vi "client.vi"() -> ()   [LabVIEW 2020]
uses:
  <vilib>/httpClient/LabVIEWHTTPClient.lvlib
panel:
  out "Output":picture
  out "Selected Image":picture
  in  "Path":path
  out "body":string
  in  "Server Address":string
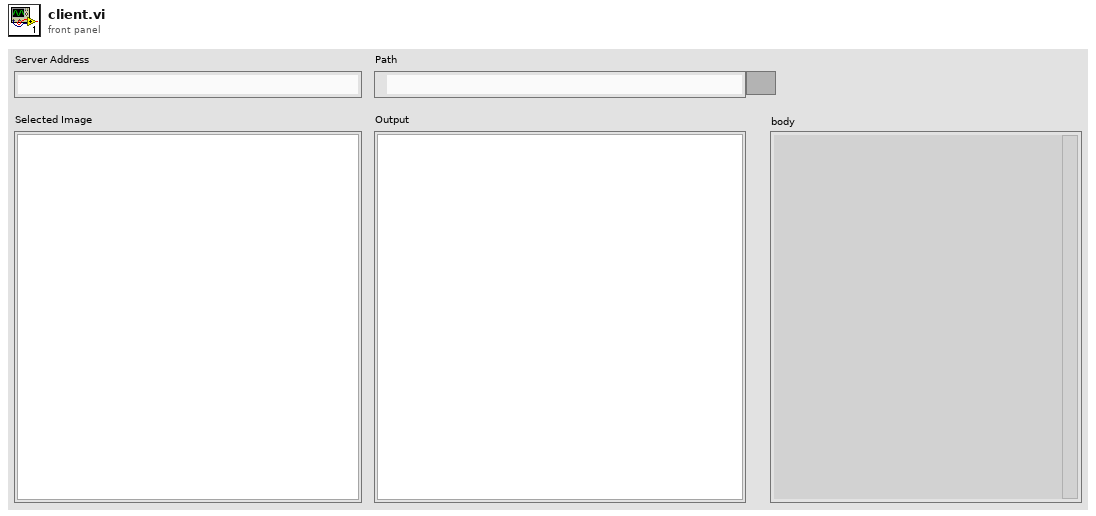
[diagram p1: front panel]
types:
  T1 = typedef "imagedata.ctl" = cluster{"image type":i32, "image depth":i32, "image":u8[], "mask":u8[], "colors":u32[], "Rectangle":cluster{"left":i16, "top":i16, "right":i16, "bottom":i16}}
  T2 = cluster{"Name":string, string, "Path":path, "name":string, string}
  T3 = cluster{"Name":string, string, "Path":path, "name":string, string}[]
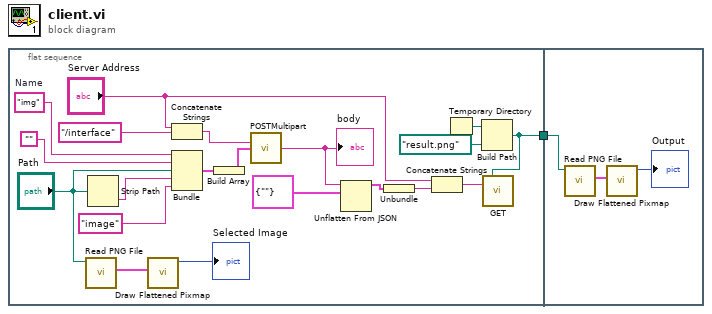
[diagram p0: block diagram]
diagram:
  n1 = flat-sequence {
    tunnel: [w3] -> w1
    tunnel: w1 -> [w22]
    frame #0 {
      w6 = "img"  # Name
      n2 = call <vilib>:"Read PNG File.vi"("path to PNG file"="Path") -> ("image data"=w14:T1)  [unwired: 8 in, 2 out]
      n3 = Strip Path(path="Path") -> (name=w10:string)  [unwired: 1 out]
      n4 = call <vilib>:"Draw Flattened Pixmap.vi"("image data"=w14) -> ("new picture"=→"Selected Image":picture)  [unwired: 8 in]
      n5 = Concatenate Strings("Server Address", "/interface") -> (w18:string)
      n6 = Bundle("Name"=w6, "", "Path"="Path", "name"=w10, "image") -> (w11:T2)  [unwired: 1 in]
      n7 = Build Array(w11) -> (w12:T3)
      n8 = call <vilib>:"POSTMultipart.vi"("url"=w18, "data"=w12) -> ("body"=w16:string)  [unwired: 10 in, 3 out]
      "body" <- w16
      n9 = Unflatten From JSON(JSON string=w16, type and defaults=cluster{"img":string} {"img"=""}) -> (value=w17:cluster{"img":string})  [unwired: 5 in, 1 out]
      n10 = Unbundle(w17) -> ("img"=w19:string)
      n11 = Concatenate Strings("Server Address", w19) -> (w21:string)
      n12 = Temporary Directory() -> (w2:path)
      n13 = Build Path(base path=w2, name or relative path=path "result.png") -> (appended path=w3:path)
      n14 = call <vilib>:"GET.vi"("output file"=w3, "url"=w21) -> ()  [unwired: 10 in, 4 out]
    }
    frame #1 {
      n15 = call <vilib>:"Read PNG File.vi"("path to PNG file"=w22) -> ("image data"=w24:T1)  [unwired: 8 in, 2 out]
      n16 = call <vilib>:"Draw Flattened Pixmap.vi"("image data"=w24) -> ("new picture"=→"Output":picture)  [unwired: 8 in]
    }
  }
